vi "Read DMD 2 Monitor Number (SubVI).vi"() -> (3 "Monitor Number":u16)   [LabVIEW 2020]
uses:
  <vilib>/Utility/config.llb/Read Key (U32).vi
  <vilib>/Utility/config.llb/Write Key (U32).vi
  <vilib>/Utility/config.llb/NI_LVConfig.lvlib
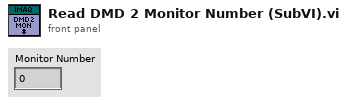
[diagram p1: front panel]
types:
  T1 = typedef "NI_LVConfig.lvlib/Config Data RefNum.ctl" = refnum<k1>
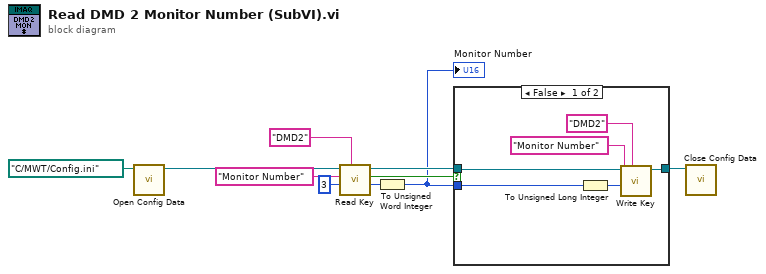
[diagram p0: block diagram]
diagram:
  n1 = call <vilib>:"Open Config Data.vi"("configuration file path"=path "C:/MWT/Config.ini") -> ("refnum"=w6:T1)  [unwired: 8 in, 2 out]
  n2 = call-poly <vilib>:"Read Key.vi"("section"="DMD2", "default value"=u32 3, "key"="Monitor Number" ("section"), "refnum"=w6) -> ("value"=w10:u32, "found?"=w4:bool, "refnum out"=w3:T1)  [unwired: 4 in, 1 out]
  n3 = To Unsigned Word Integer(number=w10) -> (unsigned 16bit integer=w1:u16)
  "Monitor Number" <- w1
  n4 = case shown="False" w4 {
    tunnel: w3 -> [w13 w17]
    tunnel: [w12 w17] -> w2
    tunnel: w1 -> [w11 _]
    frame False {
      n5 = To Unsigned Long Integer(number=w11) -> (unsigned 32bit integer=w15:u32)
      n6 = call-poly <vilib>:"Write Key.vi"("section"="DMD2", "value"=w15, "key"="Monitor Number" ("section"), "refnum"=w13) -> ("refnum out"=w12:T1)  [unwired: 5 in, 2 out]
    }
    frame True {
    }
  }
  n7 = call <vilib>:"Close Config Data.vi"("refnum"=w2) -> ()  [unwired: 9 in, 2 out]
